vi "Write OCP_Mode.vi"(8 "error in":errorcluster, 10 "OCP Mode":T1, 11 "69X_79X in":refnum<class "7976A.lvclass">) -> (0 "error out":errorcluster, 3 "69X_79X out":refnum<class "7976A.lvclass">)   [LabVIEW 2019, in "7976A.lvlib" / "7976A.lvclass"]
uses:
  Library/7976A.lvclass
  builds/Instruments/PowerSupply.lvlibp/Custom Controls/OCP Mode.ctl
  builds/Instruments/PowerSupply.lvlibp/Library/PowerSupply.lvclass
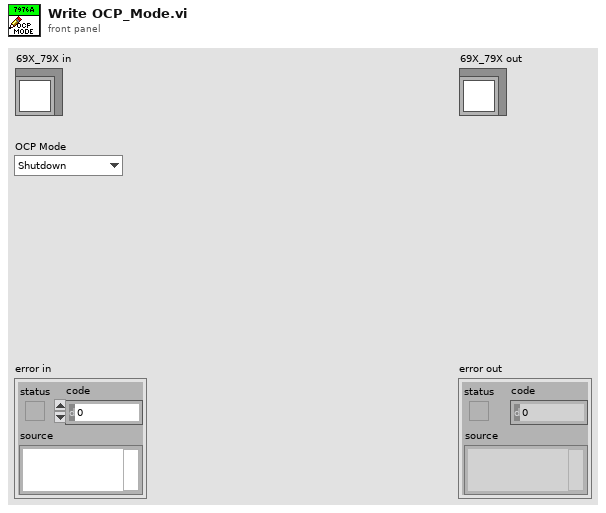
[diagram p1: front panel]
types:
  T1 = typedef "PowerSupply.lvlibp/PowerSupply.lvclass/OCP Mode.ctl" = enum16{"Shutdown", "Foldback"}
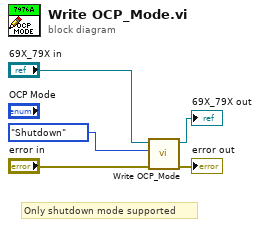
[diagram p0: block diagram]
diagram:
  # "Only shutdown mode supported"
  n1 = call-parent "Write OCP_Mode.vi"("error in"="error in", "OCP Mode"=OCP_Mode."Shutdown", "PowerSupply in"="69X_79X in") -> ("error out"=→"error out":errorcluster, "PowerSupply out"=→"69X_79X out":refnum<class "7976A.lvclass">)  [unwired: 7 in]
